vi "Template Load INI Content From File.vi"(6 "Export?":bool, 7 "FILE TO LOAD":path, 8 "error in":errorcluster, 9 "KEY":string, 10 "section":string, 11 "refnum out":T1) -> (0 "error out":errorcluster, 3 "refnum out 2":T1)   [LabVIEW 2011]
uses:
  <vilib>/Utility/config.llb/Config Data RefNum.ctl
  <vilib>/Utility/config.llb/Write Key (String).vi
  <vilib>/Utility/config.llb/NI_LVConfig.lvlib
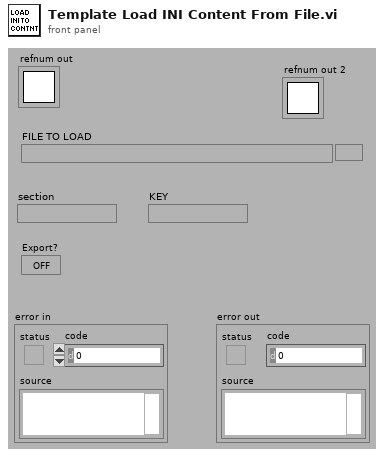
[diagram p1: front panel]
types:
  T1 = typedef "NI_LVConfig.lvlib/Config Data RefNum.ctl" = refnum<k1>
  T2 = enum16{"open", "replace", "create", "open or create", "replace or create", "replace or create with confirmation"}
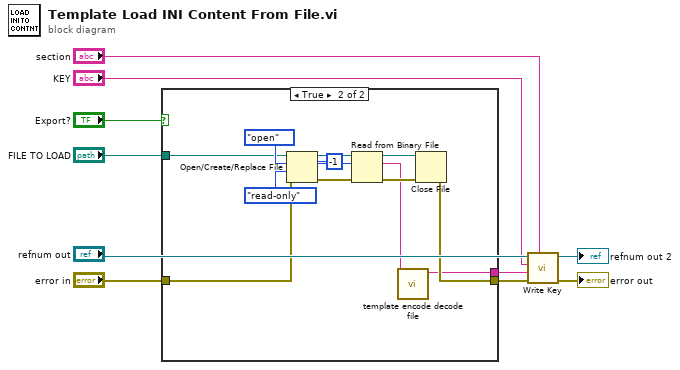
[diagram p0: block diagram]
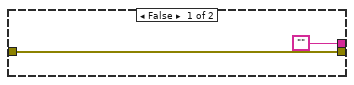
[diagram p2: hidden frame]
diagram:
  n1 = case shown="True" "Export?" {
    tunnel: "FILE TO LOAD" -> [_ w13]
    tunnel: "error in" -> [w11 w14]
    tunnel: [w11 w17] -> w8
    tunnel: ["" w15] -> w2
    frame False {
    }
    frame True {
      n2 = Open/Create/Replace File(file path (use dialog)=w13, error in=w14, operation (0:open)=T2."open", access (0:read/write)=enum16{"read/write", "read-only", "write-only"}."read-only") -> (refnum out=w23:refnum<file>, error out=w18:errorcluster)  [unwired: 3 out]
      n3 = Read from Binary File(8:w18, 10:-1 ("count"), 11:w23) -> (0:w19:errorcluster, 2:w16:string, 3:w20:refnum<file>)  [unwired: 4 out]
      n4 = call "template encode decode file.vi"("String to encode"=w16) -> ("encoded String"=w15:string)  [unwired: 1 in, 9 out]
      n5 = Close File(refnum=w20, error in=w19) -> (error out=w17:errorcluster)  [unwired: 1 out]
    }
  }
  n6 = call-poly <vilib>:"Write Key.vi"("section"="section", "error in (no error)"=w8, "value"=w2, "key"="KEY", "refnum"="refnum out") -> ("error out"=→"error out":errorcluster, "refnum out"=→"refnum out 2":T1)  [unwired: 1 in, 4 out]
